vi "Config_LoadKeys.vi"(8 "error in (no error)":errorcluster, 11 "Config In":T3) -> (0 "error out":errorcluster, 2 "output cluster":T1={"General"={"Config.ini"=path "", "Default Logging Path"=path ""}, "Hardware"={"Measure Rate (1/s)"=0, "HP DMM VISA"="", "LS 335 VISA"="", "HP DM"={"Range"=enum."Autorange", "Autozero"=FALSE, "Display"=enum."3 1/2 Digit", "Blank LCD"=FALSE}}, "Operation"={"Operation Mode"=enum."Idle-Off", "Status"="", "NewLog?"=FALSE, "OvenWarn"=FALSE}}, 3 "refnum out":T3)   [LabVIEW 2021]
uses:
  Config_Cluster.ctl
  <vilib>/Utility/config.llb/NI_LVConfig.lvlib
  <vilib>/Utility/config.llb/Read Key (Path).vi
  <vilib>/Utility/config.llb/Read Key (String).vi
  <vilib>/Utility/config.llb/Read Key (I32).vi
  Mode_Enum.ctl
  <vilib>/Utility/config.llb/Config Data RefNum.ctl
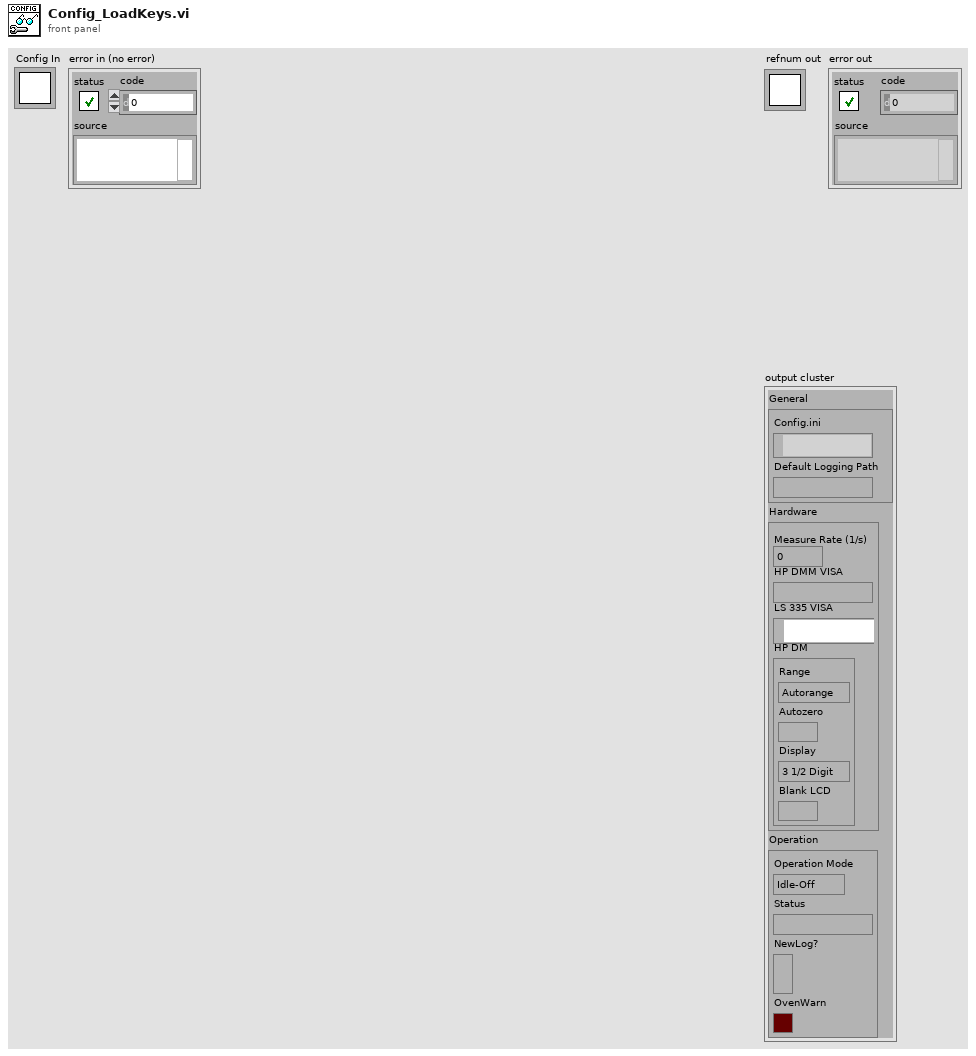
[diagram p1: front panel]
types:
  T1 = typedef "Config_Cluster.ctl" = cluster{"General":cluster{"Config.ini":path, "Default Logging Path":path}, "Hardware":cluster{"Measure Rate (1/s)":i32, "HP DMM VISA":refnum<visa-resource-name>, "LS 335 VISA":refnum<visa-resource-name>, "HP DM":cluster{"Range":enum16{"Autorange", "30mV", "300mV", "3V", "30V"}, "Autozero":bool, "Display":enum16{"3 1/2 Digit", "4 1/2 Digit", "5 1/2 Digit"}, "Blank LCD":bool}}, "Operation":cluster{"Operation Mode":T2, "Status":string, "NewLog?":bool, "OvenWarn":bool}}
  T2 = typedef "Mode_Enum.ctl" = enum16{"OvenNRDY", "Logging", "Idle-Off", "Idle"}
  T3 = typedef "NI_LVConfig.lvlib/Config Data RefNum.ctl" = refnum<k1>
  T4 = typedef "Config_Cluster.ctl" = cluster{"Hardware":cluster{"Measure Rate (1/s)":i32, "HP DMM VISA":refnum<visa-resource-name>, "LS 335 VISA":refnum<visa-resource-name>, "HP DM":cluster{"Range":enum16{"Autorange", "30mV", "300mV", "3V", "30V"}, "Autozero":bool, "Display":enum16{"3 1/2 Digit", "4 1/2 Digit", "5 1/2 Digit"}, "Blank LCD":bool}}, "Operation":cluster{"Operation Mode":T2, "Status":string, "NewLog?":bool, "OvenWarn":bool}}
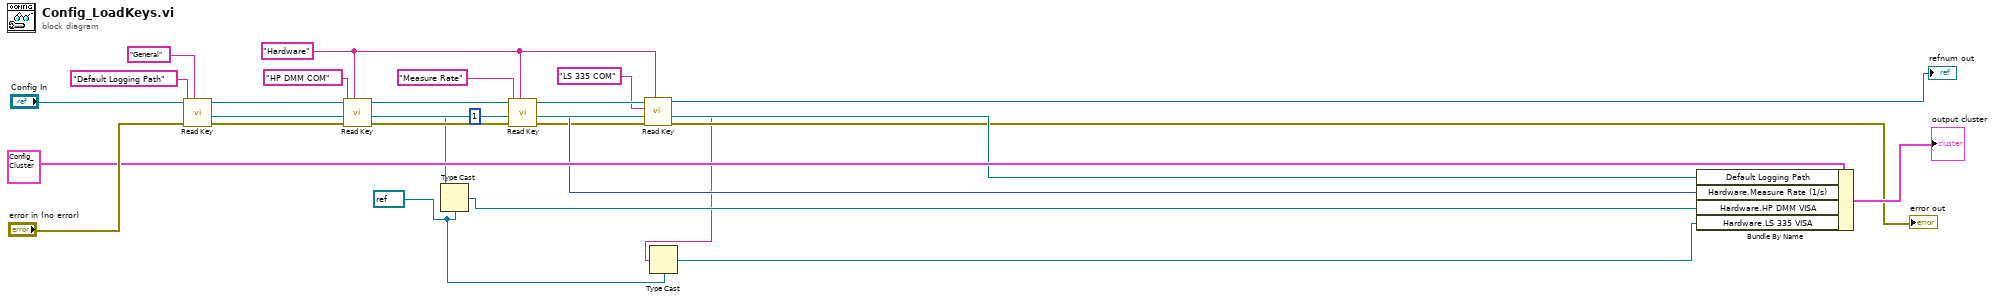
[diagram p0: block diagram]
diagram:
  w1 = refnum<visa-resource-name> refnum ("VISA resource name")
  w7 = "Hardware" ("section")
  n1 = call-poly <vilib>:"Read Key.vi"("section"="General", "error in (no error)"="error in (no error)", "key"="Default Logging Path", "refnum"="Config In") -> ("error out"=w20:errorcluster, "value"=w18:path, "refnum out"=w22:T3)  [unwired: 4 in, 1 out]
  n2 = call-poly <vilib>:"Read Key.vi"("section"=w7, "error in (no error)"=w20, "key"="HP DMM COM", "refnum"=w22) -> ("error out"=w15:errorcluster, "value"=w13:string, "refnum out"=w17:T3)  [unwired: 4 in, 1 out]
  n3 = Type Cast(type=w1, x=w13) -> (*(type *) &x=w4:refnum<visa-resource-name>)
  n4 = call-poly <vilib>:"Read Key.vi"("section"=w7, "error in (no error)"=w15, "default value"=1, "key"="Measure Rate", "refnum"=w17) -> ("error out"=w9:errorcluster, "value"=w14:i32, "refnum out"=w10:T3)  [unwired: 3 in, 1 out]
  n5 = call-poly <vilib>:"Read Key.vi"("section"=w7, "error in (no error)"=w9, "key"="LS 335 COM", "refnum"=w10) -> ("error out"=→"error out":errorcluster, "value"=w2:string, "refnum out"=→"refnum out":T3)  [unwired: 4 in, 1 out]
  n6 = Type Cast(type=w1, x=w2) -> (*(type *) &x=w3:refnum<visa-resource-name>)
  n7 = Bundle By Name(cluster=T4 {"Hardware"={"Measure Rate (1/s)"=0, "HP DMM VISA"="", "LS 335 VISA"="", "HP DM"={"Range"=enum."Autorange", "Autozero"=FALSE, "Display"=enum."3 1/2 Digit", "Blank LCD"=FALSE}}, "Operation"={"Operation Mode"=enum."Logging", "Status"="", "NewLog?"=FALSE, "OvenWarn"=FALSE}} ("Configuration Cluster"), "Default Logging Path"=w18, "Hardware.Measure Rate (1/s)"=w14, "Hardware.HP DMM VISA"=w4, "Hardware.LS 335 VISA"=w3) -> (→"output cluster":T4)
